vi "Create Synthetic Limbus Image.vi"(5 "OutLiars":bool[](array[boolean]), 7 "Array in":u8[][](array[numeric]), 8 "Direction":bool, 9 "Ofset":i32, 10 "Radiuse":i32[](array[numeric]), 11 "Centers":i32[](array[numeric])) -> (3 "Array out":u8[][](array[numeric]))   [LabVIEW 2015]
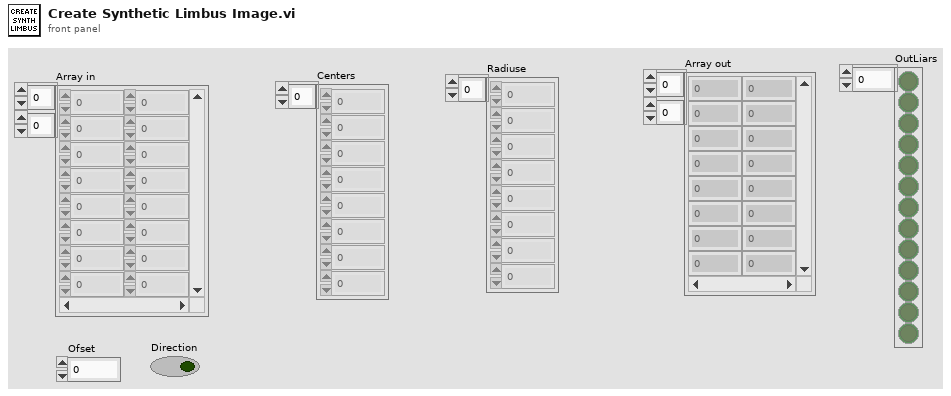
[diagram p1: front panel]
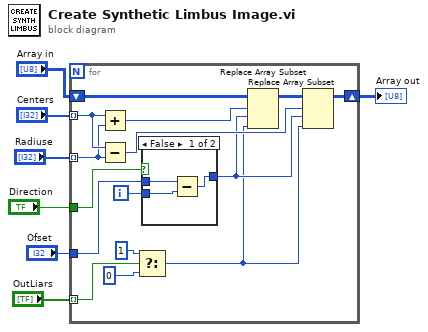
[diagram p0: block diagram]
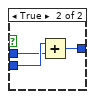
[diagram p2: hidden frame]
diagram:
  n1 = for {
    tunnel: "Centers" -> [w18] mode=indexing
    tunnel: "Radiuse" -> [w17] mode=indexing
    shift-right: [w20] -> w4
    shift-left: "Array in" -> [w22]
    tunnel: "Ofset" -> [w16]
    tunnel: "Direction" -> [w15]
    tunnel: "OutLiars" -> [w11] mode=indexing
    i -> [w19]
    n2 = Add(x=w18, y=w17) -> (x+y=w13:i32)
    n3 = Subtract(x=w18, y=w17) -> (x-y=w14:i32)
    n4 = Select(t=u8 1 ("new element/subarray"), s=w11, f=u8 0) -> (s? t:f=w9:u8)
    n5 = case shown="False" w15 {
      tunnel: w19 -> [w24 w28]
      tunnel: [w23 w27] -> w12
      tunnel: w16 -> [w25 w26]
      frame False {
        n6 = Subtract(x=w25, y=w24) -> (x-y=w23:i32)
      }
      frame True {
        n7 = Add(x=w28, y=w26) -> (x+y=w27:i32)
      }
    }
    n8 = Replace Array Subset(array=w22, new element=w9, index (row)=w13, index (col)=w12) -> (w21:u8[][])
    n9 = Replace Array Subset(array=w21, new element=w9, index (row)=w14, index (col)=w12) -> (w20:u8[][])
  }
  "Array out" <- w4
